vi "Read Command Answer.vi"(8 "error in (no error)":errorcluster, 9 "bytes to read":u32, 10 "String Seached":string, 11 "NMR in":refnum<class "NMR.lvclass">) -> (0 "error out":errorcluster, 2 "Expected Answer?":bool, 3 "NMR out":refnum<class "NMR.lvclass">)   [LabVIEW 2011, in "NMR.lvclass"]
uses:
  NMR.lvclass
  NMR.lvclass/NMR.ctl
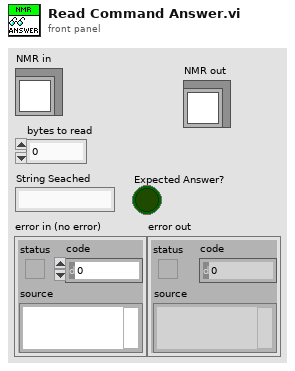
[diagram p1: front panel]
types:
  T1 = typedef "NMR.lvclass/Communication Channel.ctl" = enum16{"VISA", "DLL"}
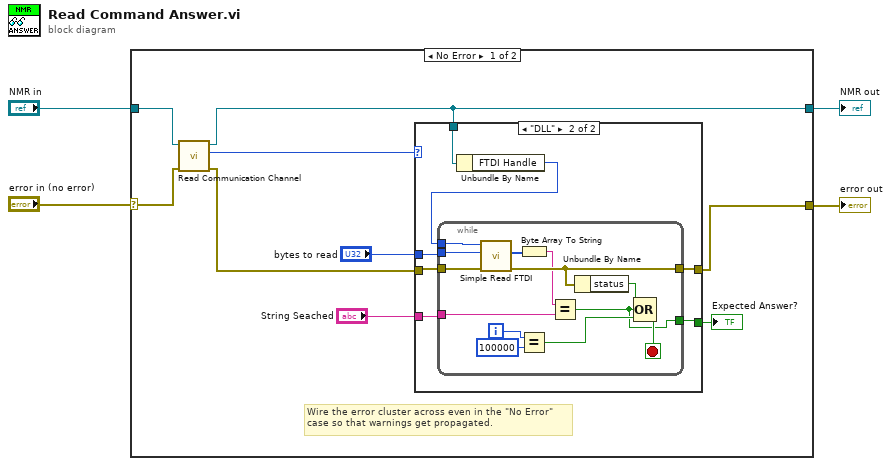
[diagram p0: block diagram]
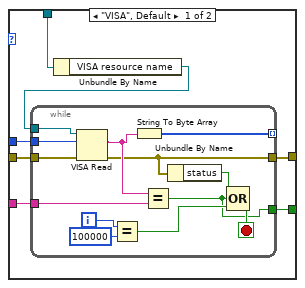
[diagram p2: hidden frame]
diagram:
  n1 = case shown="No Error" "error in (no error)" {
    selector: "error in (no error)" -> [w10 w55]
    tunnel: [w9 w55] -> w3
    tunnel: [w5 w54] -> w1
    tunnel: "NMR in" -> [w11 w54]
    frame No Error {
      # "Wire the error cluster across even in the \"No Error\"\ncase so that warnings get propagated."
      n2 = call-dynamic "Read Communication Channel.vi"("error in (no error)"=w10, "NMR in"=w11) -> ("error out"=w13:errorcluster, "Communication Channel"=w12:T1, "NMR out"=w5:refnum<class "NMR.lvclass">)  [unwired: 7 in]
      n3 = case shown="\"DLL\"" w12 {
        tunnel: w13 -> [w19 w40]
        tunnel: [w16 w34] -> w9
        tunnel: "bytes to read" -> [w18 w39]
        tunnel: "String Seached" -> [w20 w36]
        tunnel: [w17 w35] -> w6
        tunnel: w5 -> [w15 w38]
        frame "VISA", Default {
          n4 = Unbundle By Name(w15) -> ("VISA resource name"=w14:refnum<visa-resource-name>)
          n5 = while {
            tunnel: [w33] -> _ mode=indexing
            tunnel: [w27] -> w16
            tunnel: w14 -> [w26]
            tunnel: w19 -> [w25]
            tunnel: [w21] -> w17
            tunnel: w20 -> [w23]
            tunnel: w18 -> [w22]
            i -> [w32]
            stop <- w29 stop-if-true
            n6 = VISA Read(VISA resource name=w26, byte count=w22, error in (no error)=w25) -> (read buffer=w28:string, error out=w27:errorcluster)  [unwired: 2 out]
            n7 = Equal?(x=w32, y=100000) -> (x = y?=w30:bool)
            n8 = String To Byte Array(string=w28) -> (unsigned byte array=w33:u8[])
            n9 = Equal?(x=w28, y=w23) -> (x = y?=w21:bool)
            n10 = Unbundle By Name(w27) -> ("status"=w24:bool)
            n11 = Compound Arithmetic op=OR(w24, w21, w30) -> (w29:bool)
          }
        }
        frame "DLL" {
          n12 = Unbundle By Name(w38) -> ("FTDI Handle"=w37:u32)
          n13 = while {
            tunnel: [w44] -> w34
            tunnel: w40 -> [w47]
            tunnel: [w48] -> w35
            tunnel: w36 -> [w41]
            tunnel: w39 -> [w45]
            tunnel: w37 -> [w46]
            i -> [w53]
            stop <- w50 stop-if-true
            n14 = call "Simple Read FTDI.vi"("error In"=w47, "Bytes To Read"=w45, "FTDI Handle In"=w46) -> ("error out"=w44:errorcluster, "Read Data"=w43:u8[])  [unwired: 6 in, 1 out]
            n15 = Byte Array To String(unsigned byte array=w43) -> (string=w42:string)
            n16 = Equal?(x=w53, y=100000) -> (x = y?=w51:bool)
            n17 = Equal?(x=w42, y=w41) -> (x = y?=w48:bool)
            n18 = Unbundle By Name(w44) -> ("status"=w49:bool)
            n19 = Compound Arithmetic op=OR(w49, w48, w51) -> (w50:bool)
          }
        }
      }
      "Expected Answer?" <- w6
    }
    frame Error {
    }
  }
  "error out" <- w3
  "NMR out" <- w1
